vi "CheckWatchdogTimer.vi"(3 "ROS":T1, 4 "itteration":i32, 5 "LogPath in":path) -> ()   [LabVIEW 2012]
doc: "Checks the watchdog timer to close unused nodes"
uses:
  <userlib>/ROSforLV/ROS/Code/SubVIs/_ROSControl.ctl
  <userlib>/ROSforLV/ROS/Code/SubVIs/_ROSDirection.ctl
  <userlib>/ROSforLV/ROS/Code/_ROSDefinition.vi
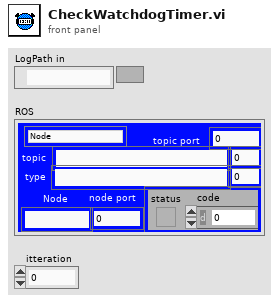
[diagram p1: front panel]
types:
  T1 = typedef "_ROSControl.ctl" = cluster{"topic port":u16, "Node":string, "topic":string, "type":string, "node port":u16, "error ":errorcluster, "Direction":T2, "Update (ms)":u16, "FIFO size":u16}
  T2 = typedef "_ROSDirection.ctl" = enum16{"Node", "Publisher", "Subscriber", "ServiceClient", "ServiceProvider"}
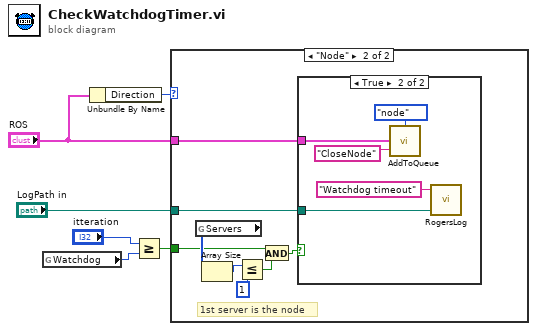
[diagram p0: block diagram]
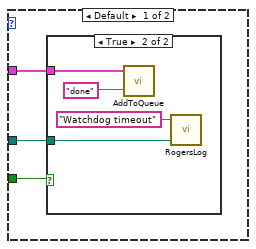
[diagram p2: hidden frame]
diagram:
  n1 = global read "_ROSDefinition.vi" "Watchdog"() -> (w3:i32)
  n2 = Unbundle By Name("ROS") -> ("Direction"=w2:T2)
  n3 = Greater Or Equal?(x="itteration", y=w3) -> (x >= y?=w5:bool)
  n4 = case shown="\"Node\"" w2 {
    tunnel: "ROS" -> [w9 w21]
    tunnel: "LogPath in" -> [w8 w20]
    tunnel: w5 -> [w7 w18]
    frame Default {
      n5 = case shown="True" w7 {
        tunnel: w8 -> [_ w12]
        tunnel: w9 -> [_ w11]
        frame False {
        }
        frame True {
          n6 = call <userlib>:"AddToQueue.vi"("Cmd"="done" ("element"), "ROS"=w11) -> ()  [unwired: 3 in, 1 out]
          n7 = call <userlib>:"RogersLog.vi"("Text to add"="Watchdog timeout", "LogPath in"=w12) -> ()  [unwired: 3 in, 2 out]
        }
      }
    }
    frame "Node" {
      # "1st server is the node"
      n8 = global read "_ROSDefinition.vi" "Servers"() -> (w19:u16[])
      n9 = Array Size(array=w19) -> (size(s)=w15:i32)
      n10 = Less Or Equal?(x=w15, y=1) -> (x <= y?=w17:bool)
      n11 = And(x=w18, y=w17) -> (x .and. y?=w16:bool)
      n12 = case shown="True" w16 {
        tunnel: w20 -> [_ w25]
        tunnel: w21 -> [_ w24]
        frame False {
        }
        frame True {
          n13 = call <userlib>:"AddToQueue.vi"("Cmd"="CloseNode" ("element"), "ROS"=w24, "Type"=enum16{"topic", "node"}."node" ("Name")) -> ()  [unwired: 2 in, 1 out]
          n14 = call <userlib>:"RogersLog.vi"("Text to add"="Watchdog timeout", "LogPath in"=w25) -> ()  [unwired: 3 in, 2 out]
        }
      }
    }
  }
